vi "dtmstodts.vi"(11 "Default in":i64) -> (3 "Numeric":dbl)   [LabVIEW 2018, in "pid-toolkit.lvlib"]
uses:
  pid-toolkit.lvlib
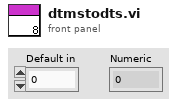
[diagram p1: front panel]
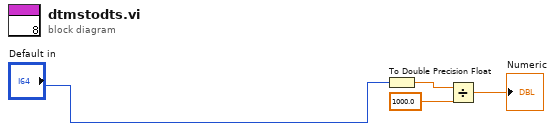
[diagram p0: block diagram]
diagram:
  n1 = To Double Precision Float(number="Default in") -> (double precision float=w1:dbl)
  n2 = Divide(x=w1, y=1000.0) -> (x/y=→"Numeric":dbl)
